vi "Close.vi"(8 "error in":errorcluster, 11 "Temperature Limit in":refnum<class "Temperature Limit.lvclass">) -> (0 "error out":errorcluster, 3 "Temperature Limit out":refnum<class "Temperature Limit.lvclass">)   [LabVIEW 2023, in "Temperature Limit.lvclass"]
uses:
  Temperature Limit.lvclass
  Parents/Limit/Limit.lvclass
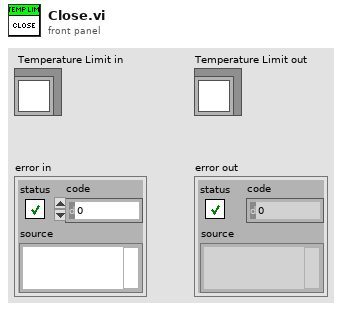
[diagram p1: front panel]
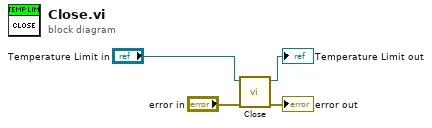
[diagram p0: block diagram]
diagram:
  n1 = call-parent "Close.vi"("error in"="error in", "Limit in"="Temperature Limit in") -> ("error out"=→"error out":errorcluster, "Limit out"=→"Temperature Limit out":refnum<class "Temperature Limit.lvclass">)  [unwired: 8 in]
